vi "Update Laser Controls.vi"(0 "cCRDS in":refnum<class "cCRDS.lvclass">, 5 "error in":errorcluster) -> (14 "cCRDS out":refnum<class "cCRDS.lvclass">, 19 "error out":errorcluster)   [LabVIEW 2015, in "cCRDS.lvclass"]
uses:
  cCRDS.lvclass
  cCRDS.lvclass/cCRDS.ctl
  <vilib>/DAQmx/read.llb/DAQmx Read (Raw 1D U16).vi
  <vilib>/DAQmx/write.llb/DAQmx Write (Digital 1D Bool NChan 1Samp 1Line).vi
  <vilib>/DAQmx/miscellaneous.llb/DAQmx Fill In Error Info.vi
  <resource>/objmgr/daqmx.rc
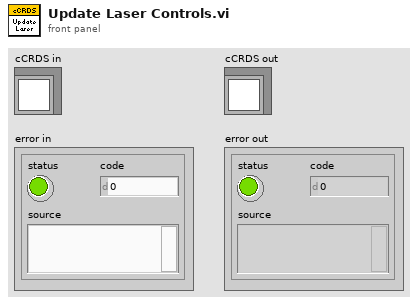
[diagram p1: front panel]
types:
  T1 = cluster{"red":bool, "Blue":bool, "Aux":bool, "Green":bool}
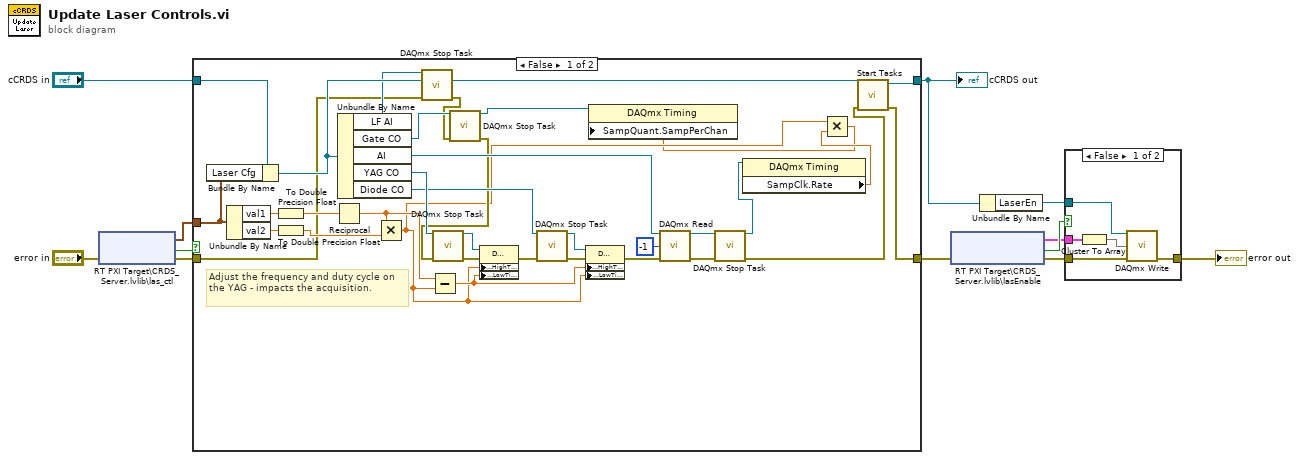
[diagram p0: block diagram]
diagram:
  n1 = shared-variable "RT PXI Target\\CRDS_Server.lvlib\\las_ctl"(error in="error in") -> (w9:cluster{"val1":sgl, "val2":sgl}, error out=w10:errorcluster, w8:bool)  [unwired: 1 in]
  n2 = case shown="False" w8 {
    tunnel: w9 -> [w29 _]
    tunnel: w10 -> [w14 w48]
    tunnel: "cCRDS in" -> [w30 w47]
    tunnel: [w16 w48] -> w3
    tunnel: [w18 w47] -> w1
    frame False {
      # "Adjust the frequency and duty cycle on the YAG - impacts the acquisition."
      n3 = Bundle By Name(cluster=w30, "Laser Cfg"=w29) -> (w19:refnum<class "cCRDS.lvclass">)
      n4 = Unbundle By Name(w29) -> ("val1"=w42:sgl, "val2"=w31:sgl)
      n5 = To Double Precision Float(number=w42) -> (double precision float=w41:dbl)
      n6 = To Double Precision Float(number=w31) -> (double precision float=w43:dbl)
      n7 = Reciprocal(x=w41) -> (1/x=w40:dbl)
      n8 = Unbundle By Name(w19) -> ("LF AI"=w15:refnum<k21>, "Gate CO"=w26:refnum<k21>, "AI"=w37:refnum<k21>, "YAG CO"=w45:refnum<k21>, "Diode CO"=w44:refnum<k21>)
      n9 = Multiply(x=w40, y=w43) -> (x*y=w22:dbl)
      n10 = call <vilib>:"DAQmx Stop Task.vi"("task/channels in"=w15, "error in"=w14) -> ("error out"=w13:errorcluster)  [unwired: 12 in, 1 out]
      n11 = Subtract(x=w40, y=w22) -> (x-y=w38:dbl)
      n12 = call <vilib>:"DAQmx Stop Task.vi"("task/channels in"=w26, "error in"=w13) -> ("task out"=w24:refnum<k21>, "error out"=w25:errorcluster)  [unwired: 12 in]
      n13 = call <vilib>:"DAQmx Stop Task.vi"("task/channels in"=w45, "error in"=w25) -> ("task out"=w39:refnum<k21>, "error out"=w33:errorcluster)  [unwired: 12 in]
      n14 = property class="DAQmx Channel"(reference=w39, error in=w33, "CO.Pulse.HighTime"=w22, "CO.Pulse.LowTime"=w38) -> (error out=w32:errorcluster)  [unwired: 1 out]
      n15 = call <vilib>:"DAQmx Stop Task.vi"("task/channels in"=w44, "error in"=w32) -> ("task out"=w46:refnum<k21>, "error out"=w34:errorcluster)  [unwired: 12 in]
      n16 = property class="DAQmx Channel"(reference=w46, error in=w34, "CO.Pulse.HighTime"=w38, "CO.Pulse.LowTime"=w22) -> (error out=w36:errorcluster)  [unwired: 1 out]
      n17 = call-poly <vilib>:"DAQmx Read.vi"("task/channels in"=w37, "number of samples per channel"=-1, "error in"=w36) -> ("task out"=w28:refnum<k21>, "error out"=w27:errorcluster)  [unwired: 10 in, 1 out]
      n18 = call <vilib>:"DAQmx Stop Task.vi"("task/channels in"=w28, "error in"=w27) -> ("task out"=w23:refnum<k21>, "error out"=w17:errorcluster)  [unwired: 12 in]
      n19 = property class="DAQmx Timing"(reference=w23) -> ("SampClk.Rate"=w21:dbl)  [unwired: 1 in, 2 out]
      n20 = Multiply(x=w22, y=w21) -> (x*y=w20:dbl)
      n21 = property class="DAQmx Timing"(reference=w24, "SampQuant.SampPerChan"=w20) -> ()  [unwired: 1 in, 2 out]
      n22 = call "Start Tasks.vi"("error in"=w17, "cCRDS in"=w19) -> ("error out"=w16:errorcluster, "cCRDS out"=w18:refnum<class "cCRDS.lvclass">)  [unwired: 8 in]
    }
    frame True {
    }
  }
  "cCRDS out" <- w1
  n23 = shared-variable "RT PXI Target\\CRDS_Server.lvlib\\lasEnable"(error in=w3) -> (w6:T1, error out=w5:errorcluster, w7:bool)  [unwired: 1 in]
  n24 = Unbundle By Name(w1) -> ("LaserEn"=w4:refnum<k21>)
  n25 = case shown="False" w7 {
    tunnel: w6 -> [w53 _]
    tunnel: w5 -> [w51 w54]
    tunnel: [w50 w54] -> w2
    tunnel: w4 -> [w49 _]
    frame False {
      n26 = Cluster To Array(cluster=w53) -> (array=w52:bool[])
      n27 = call-poly <vilib>:"DAQmx Write.vi"("task/channels in"=w49, "data"=w52, "error in"=w51) -> ("error out"=w50:errorcluster)  [unwired: 10 in, 2 out]
    }
    frame True {
    }
  }
  "error out" <- w2
